vi "workbook.create_set_description.vi"(8 "error in":errorcluster, 11 "WorkbookCreateStaging in":refnum<class "WorkbookCreateStaging.lvclass">) -> (0 "error out":errorcluster, 3 "WorkbookCreateStaging out":refnum<class "WorkbookCreateStaging.lvclass">)   [LabVIEW 2020, in "WorkbookCreateStaging.lvclass"]
doc: "Sets the description for the workbook being created, overriding the template's description."
uses:
  WorkbookCreateStaging.lvclass
  WorkbookCreateStaging.lvclass/WorkbookCreateStaging.ctl
  client.lvlib
panel:
  in  "description":string
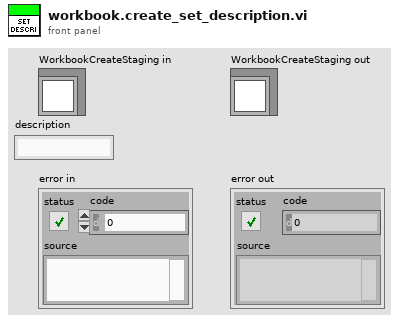
[diagram p1: front panel]
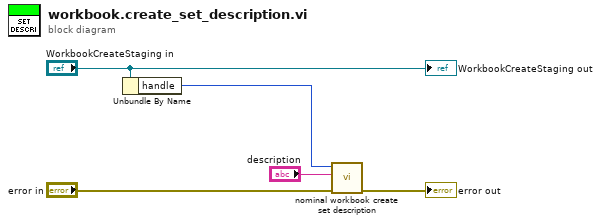
[diagram p0: block diagram]
diagram:
  n1 = Unbundle By Name("WorkbookCreateStaging in") -> ("handle"=w3:i32)
  n2 = call "nominal workbook create set description.vi"("error in (no error)"="error in", "description"="description", "staging"=w3) -> ("error out"=→"error out":errorcluster)  [unwired: 7 in, 1 out]
  "WorkbookCreateStaging out" <- "WorkbookCreateStaging in"
